vi "Append List to Report shell.vi"(6 "ordered start (1)":i32=1, 7 "ordered item type (default)":T2(ring), 8 "error in (no error)":errorcluster, 9 "list type (ordered)":enum16{"unordered", "ordered"}(ring)=enum."ordered", 10 "list elements":string[](array[string]), 11 "report in":T1) -> (0 "error out":errorcluster, 3 "report out":T1)   [LabVIEW 2020]
doc: "Adds a list of elements to the report. If you select <B>ordered</B>, the list is numbered or lettered."
uses:
  <vilib>/Utility/NIReport.llb/Generate Report Object Reference.ctl
  <vilib>/Utility/NIReport.llb/NI_report.lvclass
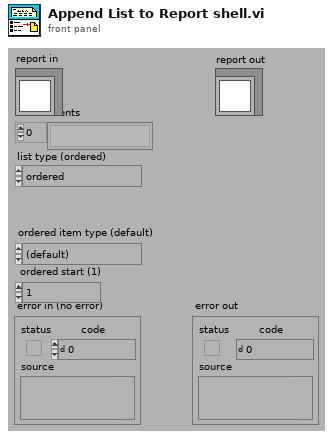
[diagram p1: front panel]
types:
  T1 = typedef "Generate Report Object Reference.ctl" = refnum<class "NI_report.lvclass">
  T2 = enum16{"(default)", "arabic numerals", "lower alpha", "upper alpha"}
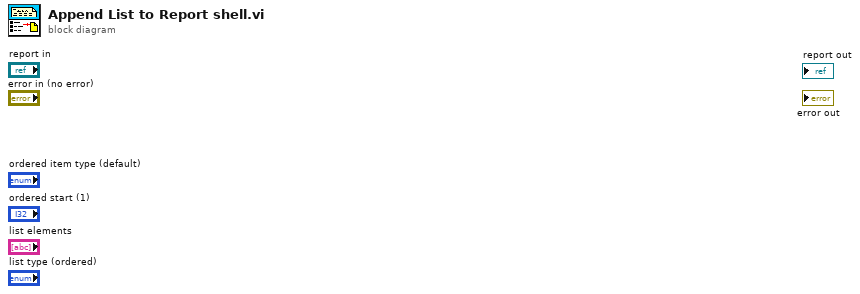
[diagram p0: block diagram]
diagram:
